vi "Build Channel Maps.vi"(8 "error in (no error)":errorcluster, 10 "Channels":string[](array[string]), 11 "Output Sequencer in":refnum<class "Output Sequencer.lvclass">) -> (0 "error out":errorcluster, 3 "Output Sequencer out":refnum<class "Output Sequencer.lvclass">)   [LabVIEW 2024, in "Output Sequencer.lvlib" / "Output Sequencer.lvclass"]
uses:
  Output Sequencer.lvclass
  Output Sequencer.lvclass/Output Sequencer.ctl
panel:
  out "'Channel' to Variable":map{string, string}(c390)
  out "Variable to Channel":map{string, string}(c390)
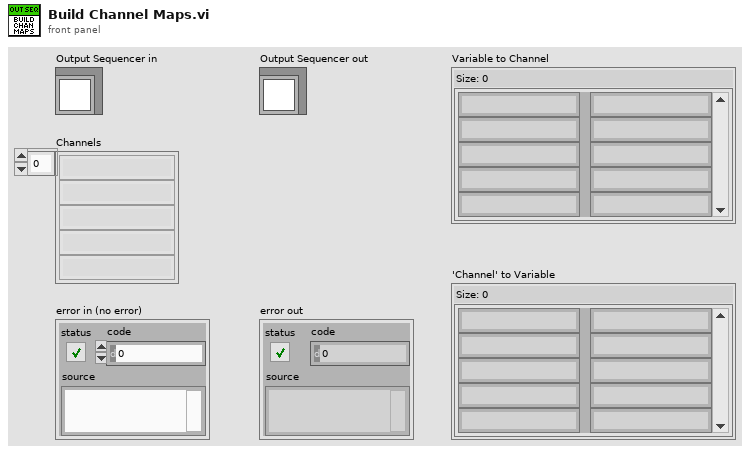
[diagram p1: front panel]
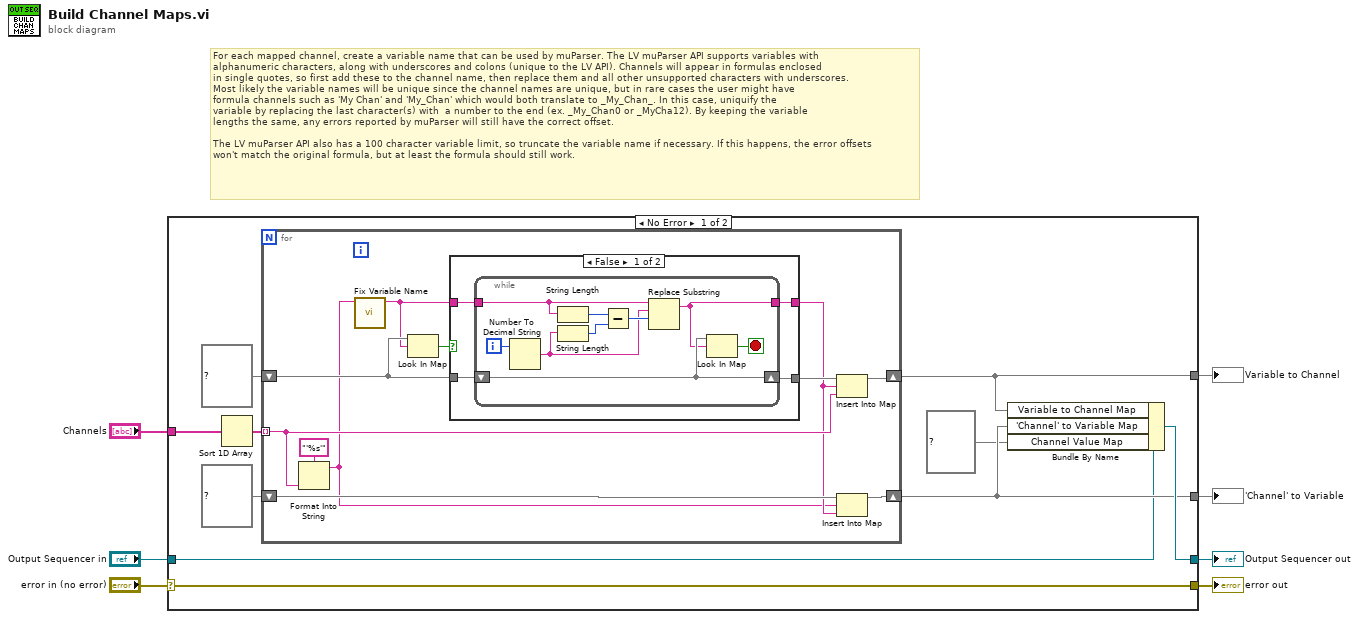
[diagram p0: block diagram]
diagram:
  # "For each mapped channel, create a variable name that can be used by muParser. The LV muParser API supports variables with\nalphanumeric characters, along with underscores and colons (unique to the LV API). Channels will appear in formulas enclosed\nin single quotes, so first add these to the channel name, then replace them and all other unsupported characters with underscores.\nMost likely the variable names will be unique since the channel names are unique, but in rare cases the user might have\nformula channels such as 'My Chan' and 'My_Chan' which would both translate to _My_Chan_. In this case, uniquify the\nvariable by replacing the last character(s) with  a number to the end (ex. _My_Chan0 or _MyCha12). By keeping the variable\nlengths the same, any errors reported by muParser will still have the correct offset.\n\nThe LV muParser API also has a 100 character variable limit, so truncate the variable name if necessary. If this happens, the error offsets\nwon't match the original formula, but at least the formula should still work."
  n1 = case shown="No Error" "error in (no error)" {
    selector: "error in (no error)" -> [w11 w45]
    tunnel: [w17 w44] -> w7
    tunnel: [w16 _] -> w6
    tunnel: [w15 _] -> w5
    tunnel: "Output Sequencer in" -> [w14 w44]
    tunnel: "Channels" -> [w13 _]
    tunnel: [w11 w45] -> w1
    frame No Error {
      n2 = Sort 1D Array(array=w13) -> (sorted array=w12:string[])
      n3 = for {
        shift-right: [w28] -> w15
        shift-left: map{string, string} {} ("Variable to Channel") -> [w23]
        shift-right: [w25] -> w16
        shift-left: map{string, string} {} ("'Channel' to Variable") -> [w27]
        tunnel: w12 -> [w21] mode=indexing
        n4 = Format Into String(format string="'%s'", w21) -> (resulting string=w19:string)  [unwired: 2 in, 1 out]
        n5 = call "Fix Variable Name.vi"("Variable in"=w19) -> ("Variable out"=w18:string)  [unwired: 10 in]
        n6 = Look In Map(map=w23, key=w18) -> (key not found?=w24:bool)  [unwired: 1 in, 1 out]
        n7 = case shown="False" w24 {
          tunnel: w23 -> [w32 w42]
          tunnel: w18 -> [w31 w43]
          tunnel: [w30 w43] -> w20
          tunnel: [w29 w42] -> w22
          frame False {
            n8 = while {
              shift-right: [w39] -> w29
              shift-left: w32 -> [w39]
              tunnel: w31 -> [w38]
              tunnel: [w34] -> w30
              i -> [w40]
              stop <- w41 stop-if-true
              n9 = Number To Decimal String(number=w40) -> (decimal integer string=w33:string)  [unwired: 1 in]
              n10 = String Length(string=w38) -> (length=w37:i32)
              n11 = String Length(string=w33) -> (length=w36:i32)
              n12 = Subtract(x=w37, y=w36) -> (x-y=w35:i32)
              n13 = Replace Substring(3:w35, 4:w33, 5:w38) -> (1:w34:string)  [unwired: 1 in, 1 out]
              n14 = Look In Map(map=w39, key=w34) -> (key not found?=w41:bool)  [unwired: 1 in, 1 out]
            }
          }
          frame True {
          }
        }
        n15 = Insert Into Map(map in=w22, key=w20, value=w21) -> (map out=w28:map{string, string})  [unwired: 2 out]
        n16 = Insert Into Map(map in=w27, key=w19, value=w20) -> (map out=w25:map{string, string})  [unwired: 2 out]
      }
      n17 = Bundle By Name(cluster=w14, "Variable to Channel Map"=w15, "'Channel' to Variable Map"=w16, "Channel Value Map"=map{string, dbl} {} ("map in")) -> (w17:refnum<class "Output Sequencer.lvclass">)
    }
    frame Error {
    }
  }
  "Output Sequencer out" <- w7
  "error out" <- w1
  "Variable to Channel" <- w5
  "'Channel' to Variable" <- w6
